vi "VariantArrayAccess.vi"   [LabVIEW 2021]
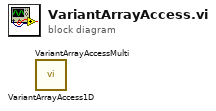
[diagram p0: block diagram]
diagram:
  n1 = call "VariantArrayAccess1D.vi"() -> ()  [unwired: 6 in, 6 out]
  n2 = call "VariantArrayAccessMulti.vi"() -> ()  [unwired: 6 in, 6 out]
